vi "Emballage_imprimerReelle.vi"(0 "path to HTML":string caption="chemin du fichier HTML", 3 "Error in":errorcluster caption="Error in (no error)") -> (10 "sortie d'erreur":errorcluster)   [LabVIEW 2020]
uses:
  Modules/FS/60_FS_Controles/60_FS_SetGet.ctl
panel:
  in  "SHDocVw.IWebBrowser2":refnum<k7>(container)
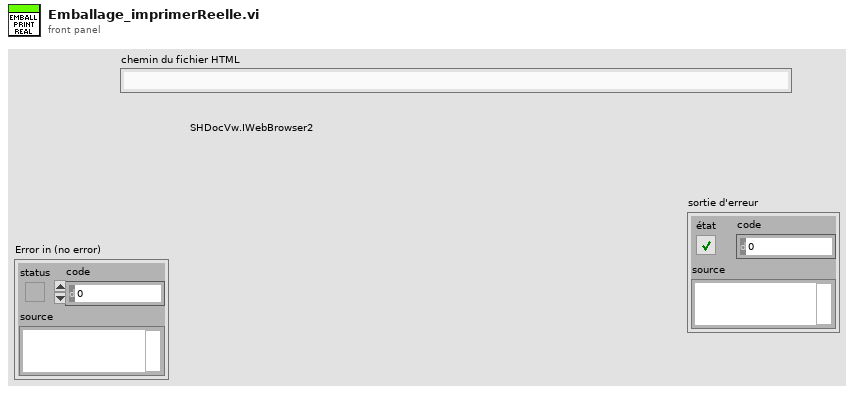
[diagram p1: front panel]
types:
  T1 = typedef "60_FS_SetGet.ctl" = enum16{"set", "get"}
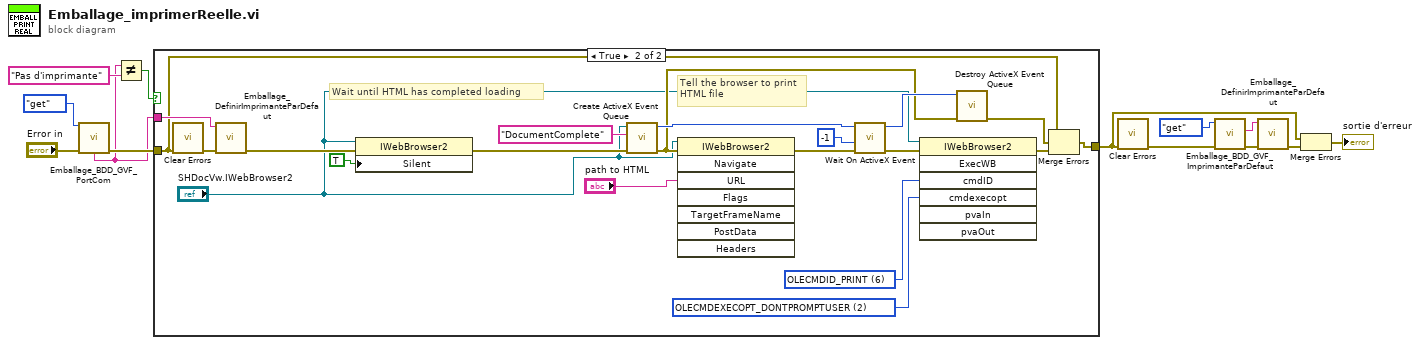
[diagram p0: block diagram]
diagram:
  n1 = call "Emballage_BDD_GVF_PortCom.vi"("Énum"=enum16{"get", "set"}."get", "Error in"="Error in") -> ("Imprimante Certif."=w1:string, "Error out"=w2:errorcluster)  [unwired: 7 in, 5 out]
  n2 = Not Equal?(x=w1, y="Pas d'imprimante") -> (x != y?=w3:bool)
  n3 = case shown="True" w3 {
    tunnel: [w14 w20] -> w7
    tunnel: w2 -> [w14 w15]
    tunnel: w1 -> [_ w19]
    frame False {
    }
    frame True {
      w33 = 2 items=["OLECMDEXECOPT_DODEFAULT", "OLECMDEXECOPT_PROMPTUSER", "OLECMDEXECOPT_DONTPROMPTUSER", "OLECMDEXECOPT_SHOWHELP"] ("cmdexecopt")
      w34 = 6 items=["OLECMDID_OPEN"=1, "OLECMDID_NEW"=2, "OLECMDID_SAVE"=3, "OLECMDID_SAVEAS"=4, "OLECMDID_SAVECOPYAS"=5, "OLECMDID_PRINT"=6, "OLECMDID_PRINTPREVIEW"=7, "OLECMDID_PAGESETUP"=8, "OLECMDID_SPELL"=9, "OLECMDID_PROPERTIES"=10, "OLECMDID_CUT"=11, "OLECMDID_COPY"=12, "OLECMDID_PASTE"=13, "OLECMDID_PASTESPECIAL"=14, "OLECMDID_UNDO"=15, "OLECMDID_REDO"=16, "OLECMDID_SELECTALL"=17, "OLECMDID_CLEARSELECTION"=18, "OLECMDID_ZOOM"=19, "OLECMDID_GETZOOMRANGE"=20, "OLECMDID_UPDATECOMMANDS"=21, "OLECMDID_REFRESH"=22, "OLECMDID_STOP"=23, "OLECMDID_HIDETOOLBARS"=24, "OLECMDID_SETPROGRESSMAX"=25, "OLECMDID_SETPROGRESSPOS"=26, "OLECMDID_SETPROGRESSTEXT"=27, "OLECMDID_SETTITLE"=28, "OLECMDID_SETDOWNLOADSTATE"=29, "OLECMDID_STOPDOWNLOAD"=30, "OLECMDID_ONTOOLBARACTIVATED"=31, "OLECMDID_FIND"=32, "OLECMDID_DELETE"=33, "OLECMDID_HTTPEQUIV"=34, "OLECMDID_HTTPEQUIV_DONE"=35, "OLECMDID_ENABLE_INTERACTION"=36, "OLECMDID_ONUNLOAD"=37, "OLECMDID_PROPERTYBAG2"=38, "OLECMDID_PREREFRESH"=39, "OLECMDID_SHOWSCRIPTERROR"=40, "OLECMDID_SHOWMESSAGE"=41, "OLECMDID_SHOWFIND"=42, "OLECMDID_SHOWPAGESETUP"=43, "OLECMDID_SHOWPRINT"=44, "OLECMDID_CLOSE"=45, "OLECMDID_ALLOWUILESSSAVEAS"=46, "OLECMDID_DONTDOWNLOADCSS"=47] ("cmdID")
      # "Tell the browser to print\nHTML file"
      # "Wait until HTML has completed loading"
      n4 = call <vilib>:"Clear Errors.vi"("error in (no error)"=w15) -> ("error out"=w16:errorcluster)  [unwired: 5 in, 1 out]
      n5 = call "Emballage_DefinirImprimanteParDefaut.vi"("Error in"=w16, "Imprimante"=w19) -> ("Error out"=w18:errorcluster)  [unwired: 9 in]
      n6 = property class="IWebBrowser2"(reference="SHDocVw.IWebBrowser2", error in=w18, "Silent"=TRUE) -> (error out=w26:errorcluster)  [unwired: 1 out]
      n7 = call <vilib>:"Create ActiveX Event Queue.vi"("error in (no error)"=w26, "Event Name"="DocumentComplete", "Automation Refnum"="SHDocVw.IWebBrowser2") -> ("error out"=w24:errorcluster, "Event Queue"=w31:i32)  [unwired: 1 in, 2 out]
      n8 = invoke class="IWebBrowser2" method="Navigate"(reference="SHDocVw.IWebBrowser2", error in=w24, "URL"="path to HTML") -> (error out=w25:errorcluster)  [unwired: 5 in, 7 out]
      n9 = call <vilib>:"Wait On ActiveX Event.vi"("error in (no error)"=w25, "ms Timeout (-1)"=-1 ("ms timeout (-1)"), "Event Queue"=w31) -> ("error out"=w23:errorcluster, "Event Queue Out"=w30:i32)  [unwired: 1 in, 2 out]
      n10 = invoke class="IWebBrowser2" method="ExecWB"(reference="SHDocVw.IWebBrowser2", error in=w23, "cmdID"=w34, "cmdexecopt"=w33) -> (error out=w21:errorcluster)  [unwired: 3 in, 6 out]
      n11 = call <vilib>:"Destroy ActiveX Event Queue.vi"("error in (no error)"=w24, "Event Queue"=w30) -> ("error out"=w22:errorcluster)  [unwired: 5 out]
      n12 = Merge Errors(w15, w22, w21) -> (w20:errorcluster)
    }
  }
  n13 = call <vilib>:"Clear Errors.vi"("error in (no error)"=w7) -> ("error out"=w11:errorcluster)  [unwired: 5 in, 1 out]
  n14 = call "Emballage_BDD_GVF_ImprimanteParDefaut.vi"("Error in"=w11, "SetGet"=60_FS_SetGet."get") -> ("Error out"=w10:errorcluster, "Imprimante Par defaut"=w9:string)  [unwired: 8 in]
  n15 = call "Emballage_DefinirImprimanteParDefaut.vi"("Error in"=w10, "Imprimante"=w9) -> ("Error out"=w6:errorcluster)  [unwired: 9 in]
  n16 = Merge Errors(w7, w6) -> (→"sortie d'erreur":errorcluster)
